vi "Update Pump State.vi"(6 "Sender":refnum<class "Sender.lvclass">, 10 "Pump State":bool, 11 "TEMPLATE Actor in":refnum<class "TEMPLATE Actor.lvclass">) -> (0 "Error out":errorcluster, 3 "TEMPLATE Actor out":refnum<class "TEMPLATE Actor.lvclass">)   [LabVIEW 2025, in "TEMPLATE Actor.lvlib" / "TEMPLATE Actor.lvclass"]
uses:
  TEMPLATE Actor.lvclass
  <vilib>/Nathan Davis/jettl/jettl/jettl/Sender/Sender/Sender.lvclass
  TEMPLATE Actor.lvclass/TEMPLATE Actor.ctl
  Update Pump State Msg/Decorator.vi
  Update Pump State Msg/Update Pump State Msg.lvlib
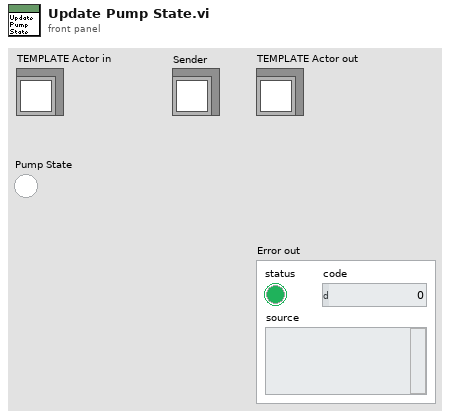
[diagram p1: front panel]
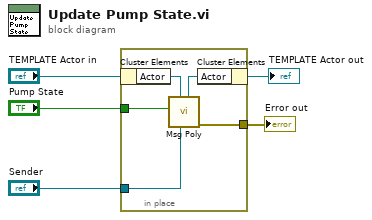
[diagram p0: block diagram]
diagram:
  n1 = in-place {
    in-place-border: [w8] -> w1
    in-place-border: "Sender" -> [w6]
    in-place-border: "Pump State" -> [w7]
    n2 = in-place-cluster #1("TEMPLATE Actor in") -> ("Actor"=w10:refnum<class "Actor.lvclass">)
    n3 = call-poly "Msg Poly.vi"("Sender"=w6, "Actor in"=w10, "Pump State"=w7) -> ("Error out"=w8:errorcluster, "Actor out"=w9:refnum<class "Actor.lvclass">)  [unwired: 7 in]
    n4 = in-place-cluster #1("Actor"=w9) -> (→"TEMPLATE Actor out":refnum<class "TEMPLATE Actor.lvclass">)
  }
  "Error out" <- w1
